vi "Initialize TCP Refs.vi"(8 "error in (no error)":errorcluster, 11 "Name":string) -> (0 "error out":errorcluster, 3 "TCP Refs":T1)   [LabVIEW 2015, in "Instrument Addon Engine.lvlib" / "Network Common API.lvlib"]
uses:
  Network Common API.lvlib
  TCP Refs.ctl
  Network Comm Global Ref.ctl
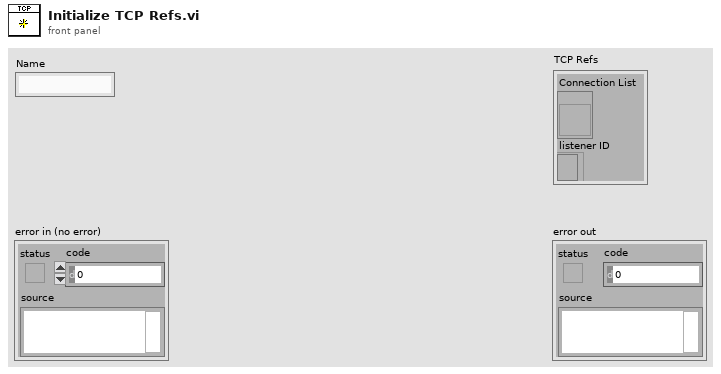
[diagram p1: front panel]
types:
  T1 = typedef "Instrument Addon Engine.lvlib/Network Common API.lvlib/TCP Refs.ctl" = cluster{"Connection List":T2, "listener ID":refnum<k5>}
  T2 = typedef "Instrument Addon Engine.lvlib/Network Common API.lvlib/Network Comm Global Ref.ctl" = refnum<vi>
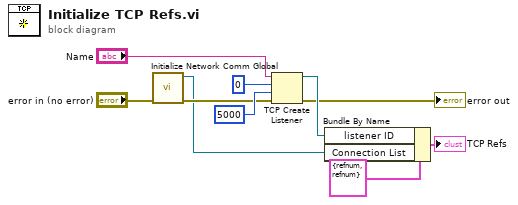
[diagram p0: block diagram]
diagram:
  n1 = call "Initialize Network Comm Global.vi"("error in (no error)"="error in (no error)") -> ("error out"=w7:errorcluster, "Ref"=w3:T2)  [unwired: 9 in]
  n2 = TCP Create Listener(8:w7, 9:5000 ("timeout ms (25000)"), 10:u16 0 ("port"), 11:"Name") -> (0:→"error out":errorcluster, 3:w10:refnum<k5>)  [unwired: 1 in, 1 out]
  n3 = Bundle By Name(cluster=T1 {"Connection List"=refnum, "listener ID"=refnum} ("TCP Refs"), "listener ID"=w10, "Connection List"=w3) -> (→"TCP Refs":T1)
